vi "GLIMPSE fetch TTB value.vi"(5 "Array of TTB Values (ms)":u32[](array[numeric]), 7 "Logical Frame Number\n(starting with zero)":u32) -> (0 "Array index":u32, 1 "TTB value out":u32)   [LabVIEW 2016]
uses:
  GLIMPSE Globals.vi
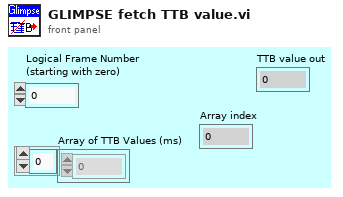
[diagram p1: front panel]
types:
  T1 = enum16{"Frames", "Fields, Odd 1st", "Fields, Even 1st", "Fields, Averaged"}
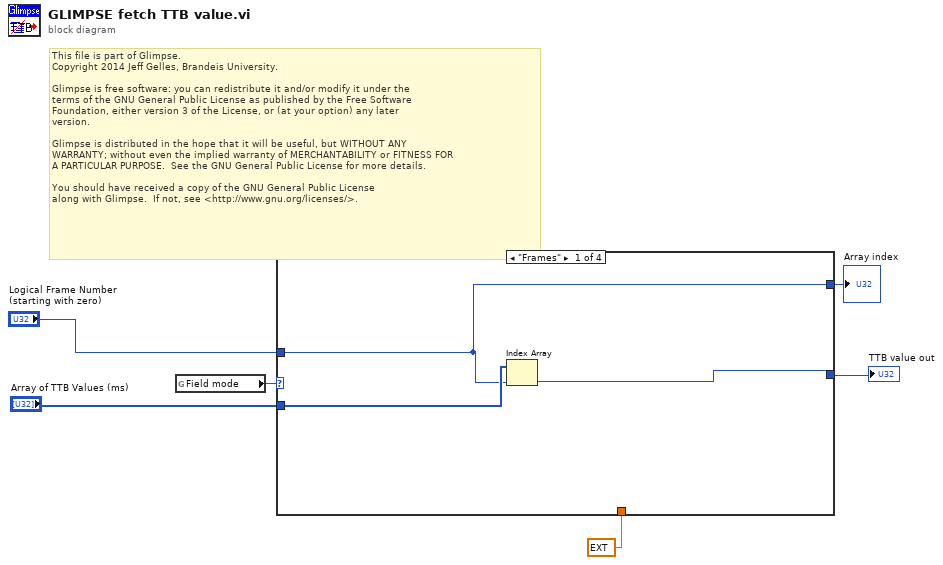
[diagram p0: block diagram]
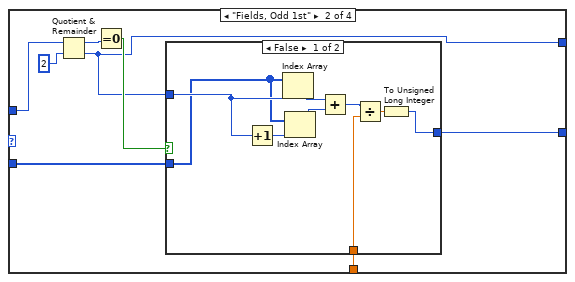
[diagram p2: hidden frame]
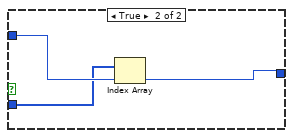
[diagram p3: hidden frame]
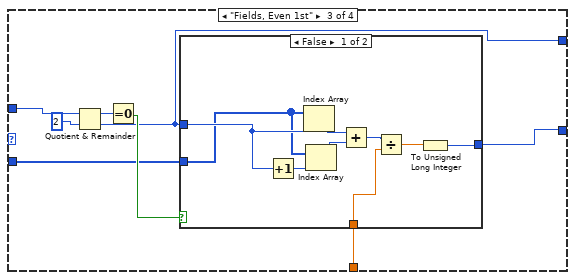
[diagram p4: hidden frame]
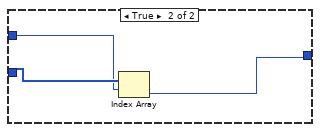
[diagram p5: hidden frame]
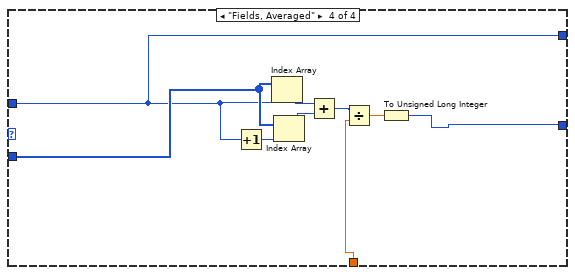
[diagram p6: hidden frame]
diagram:
  # "This file is part of Glimpse. \nCopyright 2014 Jeff Gelles, Brandeis University.    \n\nGlimpse is free software: you can redistribute it and/or modify it under the \nterms of the GNU General Public License as published by the Free Software \nFoundation, either version 3 of the License, or (at your option) any later \nversion.\n\nGlimpse is distributed in the hope that it will be useful, but WITHOUT ANY \nWARRANTY; without even the implied warranty of MERCHANTABILITY or FITNESS FOR \nA PARTICULAR PURPOSE.  See the GNU General Public License for more details.\n\nYou should have received a copy of the GNU General Public License\nalong with Glimpse.  If not, see <http://www.gnu.org/licenses/>."
  n1 = global read "GLIMPSE Globals.vi" "Field mode"() -> (w3:T1)
  n2 = case shown="\"Frames\"" w3 {
    tunnel: "Array of TTB Values (ms)" -> [w9 w13 w33 w54]
    tunnel: "Logical Frame Number\n(starting with zero)" -> [w7 w16 w36 w50]
    tunnel: [w8 w11 w32 w52] -> w6
    tunnel: ext 2.0 ("y") -> [_ w12 w31 w51]
    tunnel: [w7 w10 w30 w50] -> w1
    frame "Frames" {
      n3 = Index Array(array=w9, index=w7) -> (element=w8:u32)
    }
    frame "Fields, Odd 1st" {
      n4 = Quotient & Remainder(x=w16, y=u32 2) -> (x-y*floor(x/y)=w15:u32, floor(x/y)=w10:u32)
      n5 = Equal To 0?(x=w15) -> (x = 0?=w14:bool)
      n6 = case shown="False" w14 {
        tunnel: w10 -> [w22 w29]
        tunnel: w13 -> [w21 w28]
        tunnel: [w19 w27] -> w11
        tunnel: w12 -> [w20 _]
        frame False {
          n7 = Increment(x=w22) -> (x+1=w26:u32)
          n8 = Index Array(array=w21, index=w22) -> (element=w25:u32)
          n9 = Index Array(array=w21, index=w26) -> (element=w24:u32)
          n10 = Add(x=w25, y=w24) -> (x+y=w23:u32)
          n11 = Divide(x=w23, y=w20) -> (x/y=w18:ext)
          n12 = To Unsigned Long Integer(number=w18) -> (unsigned 32bit integer=w19:u32)
        }
        frame True {
          n13 = Index Array(array=w28, index=w29) -> (element=w27:u32)
        }
      }
    }
    frame "Fields, Even 1st" {
      n14 = Quotient & Remainder(x=w36, y=u32 2) -> (x-y*floor(x/y)=w35:u32, floor(x/y)=w30:u32)
      n15 = Equal To 0?(x=w35) -> (x = 0?=w34:bool)
      n16 = case shown="False" w34 {
        tunnel: w30 -> [w42 w48]
        tunnel: w33 -> [w41 w49]
        tunnel: [w39 w47] -> w32
        tunnel: w31 -> [w38 _]
        frame False {
          n17 = Increment(x=w42) -> (x+1=w46:u32)
          n18 = Index Array(array=w41, index=w42) -> (element=w45:u32)
          n19 = Index Array(array=w41, index=w46) -> (element=w44:u32)
          n20 = Add(x=w45, y=w44) -> (x+y=w43:u32)
          n21 = Divide(x=w43, y=w38) -> (x/y=w40:ext)
          n22 = To Unsigned Long Integer(number=w40) -> (unsigned 32bit integer=w39:u32)
        }
        frame True {
          n23 = Index Array(array=w49, index=w48) -> (element=w47:u32)
        }
      }
    }
    frame "Fields, Averaged" {
      n24 = Increment(x=w50) -> (x+1=w58:u32)
      n25 = Index Array(array=w54, index=w50) -> (element=w57:u32)
      n26 = Index Array(array=w54, index=w58) -> (element=w56:u32)
      n27 = Add(x=w57, y=w56) -> (x+y=w55:u32)
      n28 = Divide(x=w55, y=w51) -> (x/y=w53:ext)
      n29 = To Unsigned Long Integer(number=w53) -> (unsigned 32bit integer=w52:u32)
    }
  }
  "TTB value out" <- w6
  "Array index" <- w1
